vi "Display and Log Errors.vi"() -> ()   [LabVIEW 2015, in "Diagnostics Addon Engine.lvlib"]
uses:
  Diagnostics Addon Engine.lvlib
  SubVIs/Error Handling API/Print/Display and Log Custom Device Error.vi
  <vilib>/NI Veristand/Custom Device Tools/Custom Device Utility Library/NI VeriStand - Print Debug String.vi
  SubVIs/Error Handling API/Error Handling API.lvlib
  SubVIs/Inline Async API/Inline Async API.lvlib
panel:
  in  "Parent":string
  in  "Parameters":string
  in  "stop":bool
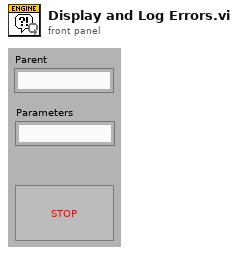
[diagram p1: front panel]
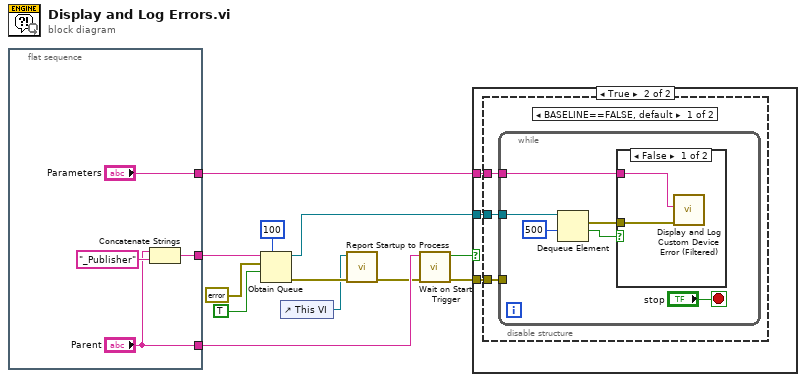
[diagram p0: block diagram]
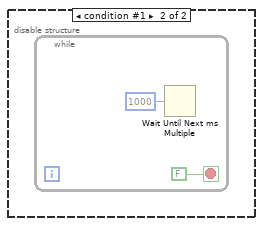
[diagram p4: hidden frame]
diagram:
  n1 = flat-sequence {
    tunnel: ["Parameters"] -> w9
    tunnel: [w14] -> w8
    tunnel: ["Parent"] -> w6
    frame #0 {
      n2 = Concatenate Strings("Parent", "_Publisher" ("name (unnamed)")) -> (w14:string)
    }
  }
  n3 = Obtain Queue(max queue size (-1, unlimited)=100, name (unnamed)=w8, element data type=errorcluster {"status"=FALSE, "code"=0, "source"=""} ("element"), create if not found? (T)=TRUE) -> (queue out=w10:refnum<queue>, error out=w5:errorcluster)  [unwired: 1 in, 1 out]
  n4 = control-ref of="This VI"() -> (w3:refnum<vi>)
  n5 = call "Report Startup to Process.vi"("Error"=w5, "This VI"=w3) -> ("error out"=w4:errorcluster)  [unwired: 9 in]
  n6 = call "Wait on Start Trigger.vi"("error in (no error)"=w4, "Name"=w6) -> ("error out"=w2:errorcluster, "notification"=w1:bool)  [unwired: 8 in]
  n7 = case shown="True" w1 {
    tunnel: w10 -> [_ w19]
    tunnel: w9 -> [_ w18]
    tunnel: w2 -> [_ w17]
    frame False {
    }
    frame True {
      n8 = disable-structure shown="BASELINE==FALSE, default" {
        disable-tunnel: w19 -> [w22 _]
        disable-tunnel: w18 -> [w21 _]
        disable-tunnel: w17 -> [w20 _]
        frame condition #0 (active) {
          n9 = while {
            tunnel: w22 -> [w28]
            tunnel: w21 -> [w27]
            tunnel: w20 -> [_]
            stop <- "stop" stop-if-true
            n10 = Dequeue Element(queue=w28, timeout in ms (-1)=500) -> (element=w26:errorcluster, timed out?=w24:bool)  [unwired: 1 in, 2 out]
            n11 = case shown="False" w24 {
              tunnel: w26 -> [w30 _]
              tunnel: w27 -> [w29 _]
              frame False {
                n12 = call "Display and Log Custom Device Error (Filtered).vi"("error in (no error)"=w30, "Your code's public name"=w29) -> ()  [unwired: 10 in]
              }
              frame True {
              }
            }
          }
        }
        frame condition #1 {
          n13 = while {
            stop <- FALSE stop-if-true
            n14 = Wait Until Next ms Multiple(millisecond multiple=u32 1000) -> ()  [unwired: 1 out]
          }
        }
      }
    }
  }
